vi "Event Handle Loop_Stop.vi"(8 "error in (no error)":errorcluster, 11 "QTab Class in":refnum<class "QTab Class.lvclass">) -> (0 "error out":errorcluster, 3 "QTab Class out":refnum<class "QTab Class.lvclass">)   [LabVIEW 2020, in "QTab.lvlib" / "QTab Class.lvclass"]
uses:
  QTab Class.lvclass
  QTab Class.lvclass/QTab Class.ctl
  QMenu Class/QMenu Class.lvclass
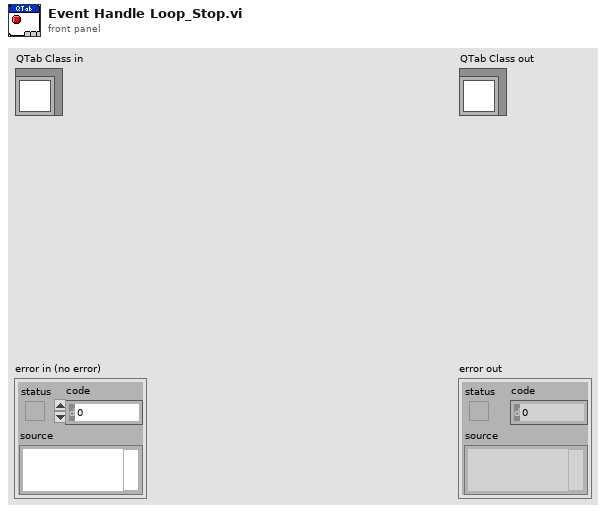
[diagram p1: front panel]
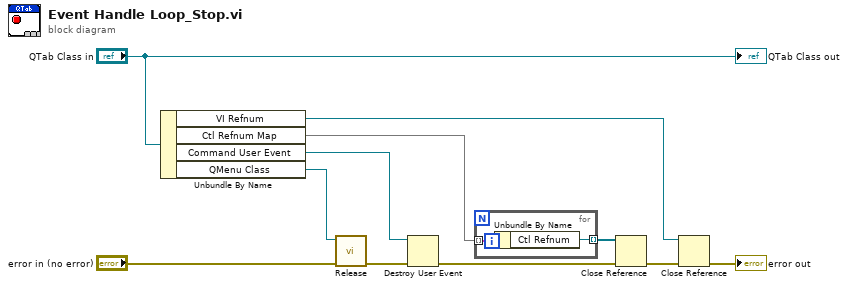
[diagram p0: block diagram]
diagram:
  n1 = Unbundle By Name("QTab Class in") -> ("VI Refnum"=w6:refnum<vi>, "Ctl Refnum Map"=w9:map{string, refnum<vi>}, "Command User Event"=w10:refnum<user-event>, "QMenu Class"=w2:refnum<class "QMenu Class.lvclass">)
  n2 = call "Release.vi"("error in (no error)"="error in (no error)", "QMenu Class in"=w2) -> ("error out"=w3:errorcluster)  [unwired: 9 in]
  n3 = Destroy User Event(user event=w10, error in=w3) -> (error out=w4:errorcluster)
  n4 = for {
    tunnel: w9 -> [w13] mode=indexing
    tunnel: [w12] -> w8 mode=indexing
    n5 = Unbundle By Name(w13) -> ("Ctl Refnum"=w12:refnum<vi>)
  }
  n6 = Close Reference(reference=w8, error in (no error)=w4) -> (error out=w7:errorcluster)
  n7 = Close Reference(reference=w6, error in (no error)=w7) -> (error out=→"error out":errorcluster)
  "QTab Class out" <- "QTab Class in"
